vi "serial_work_Init.vi"(0 "object in":refnum<class "serial_work.lvclass">, 5 "error in (no error)":errorcluster) -> (14 "object out":refnum<class "serial_work.lvclass">, 19 "error out":errorcluster)   [LabVIEW 2016, in "serial_work.lvclass"]
uses:
  serial_work.lvclass
  serial_work.lvclass/serial_work.ctl
  tcp_work_class/tcp_work.lvclass
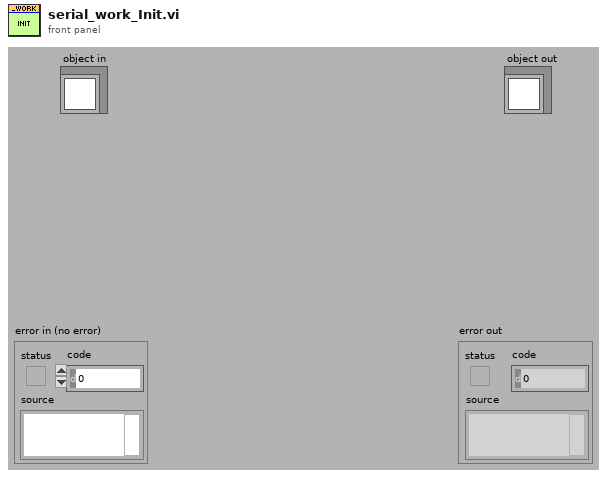
[diagram p1: front panel]
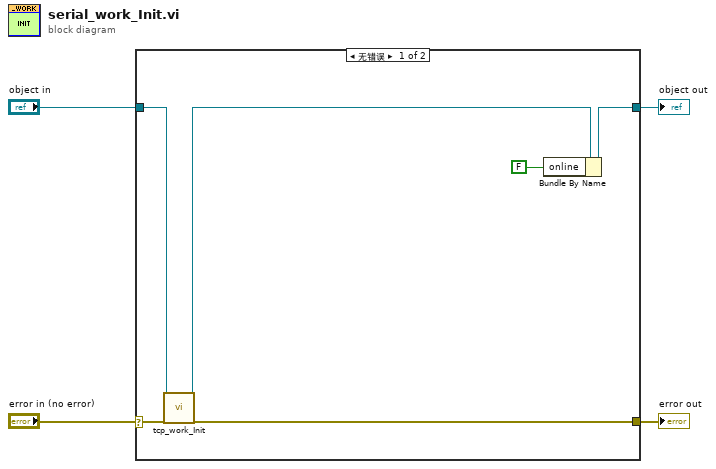
[diagram p0: block diagram]
diagram:
  n1 = case shown="无错误" "error in (no error)" {
    selector: "error in (no error)" -> [w8 w11]
    tunnel: [w10 w12] -> w4
    tunnel: "object in" -> [w6 w12]
    tunnel: [w7 w11] -> w1
    frame No Error {
      n2 = call "tcp_work_Init.vi"("object in"=w6, "error in (no error)"=w8) -> ("object out"=w5:refnum<class "serial_work.lvclass">, "error out"=w7:errorcluster)  [unwired: 16 in]
      n3 = Bundle By Name(cluster=w5, "online"=FALSE ("None")) -> (w10:refnum<class "serial_work.lvclass">)
    }
    frame Error {
    }
  }
  "object out" <- w4
  "error out" <- w1
